vi "Launch.vi"   [LabVIEW 2020, in "AR Example.lvlib"]
uses:
  AR Example.lvlib
  UI/UI.vi
  UI/UI.lvclass
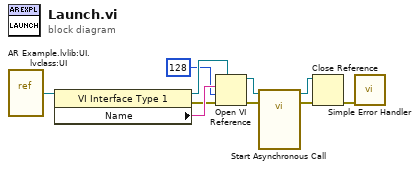
[diagram p0: block diagram]
diagram:
  n1 = vi-ref "AR Example.lvlib:UI.lvclass:UI.vi"() -> (w10:refnum<vi>)
  n2 = property class="VI Interface Type 1"(reference=w10) -> (reference out=w6:refnum<vi>, error out=w3:errorcluster, "Name"=w9:string)  [unwired: 1 in]
  n3 = Open VI Reference(type specifier VI Refnum (for type only)=w6, vi path=w9, options=128, error in (no error)=w3) -> (vi reference=w8:refnum<vi>, error out=w7:errorcluster)  [unwired: 2 in]
  n4 = call-by-ref "Start Asynchronous Call"(reference=w8, error in=w7) -> (reference out=w4:refnum<vi>, error out=w5:errorcluster)  [unwired: 12 in]
  n5 = Close Reference(reference=w4, error in (no error)=w5) -> (error out=w2:errorcluster)
  n6 = call <vilib>:"Simple Error Handler.vi"("error in (no error)"=w2) -> ()  [unwired: 4 in, 5 out]
